vi "Labview Hardware Config file read key.vi"(5 "error in (no error)":errorcluster, 6 "Interactive?":bool=TRUE, 7 "key name in":string="Port", 8 "section":string="Panasonic AG7300") -> (0 "error out":errorcluster, 1 "File read":path, 3 "key vlue out":string)   [LabVIEW 2016]
uses:
  <vilib>/Utility/config.llb/NI_LVConfig.lvlib
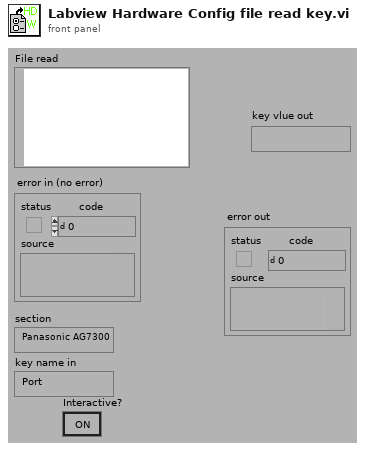
[diagram p1: front panel]
types:
  T1 = typedef "NI_LVConfig.lvlib/Config Data RefNum.ctl" = refnum<k1>
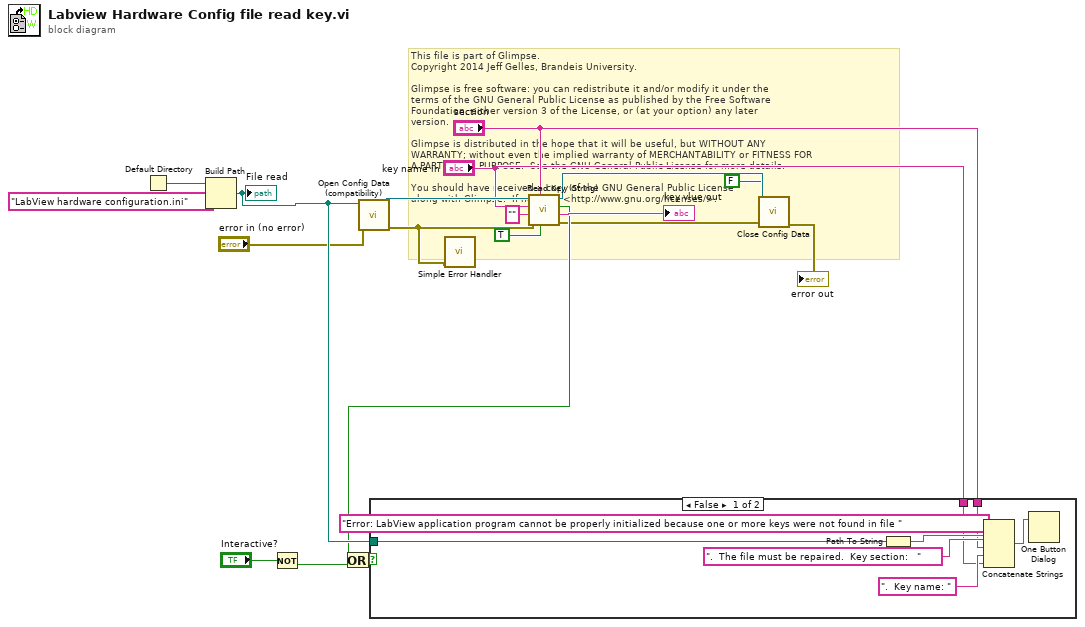
[diagram p0: block diagram]
diagram:
  # "This file is part of Glimpse. \nCopyright 2014 Jeff Gelles, Brandeis University.    \n\nGlimpse is free software: you can redistribute it and/or modify it under the \nterms of the GNU General Public License as published by the Free Software \nFoundation, either version 3 of the License, or (at your option) any later \nversion.\n\nGlimpse is distributed in the hope that it will be useful, but WITHOUT ANY \nWARRANTY; without even the implied warranty of MERCHANTABILITY or FITNESS FOR \nA PARTICULAR PURPOSE.  See the GNU General Public License for more details.\n\nYou should have received a copy of the GNU General Public License\nalong with Glimpse.  If not, see <http://www.gnu.org/licenses/>."
  n1 = Default Directory() -> (w18:path)
  n2 = Build Path(base path=w18, name or relative path="LabView hardware configuration.ini") -> (appended path=w15:path)
  "File read" <- w15
  n3 = Not(x="Interactive?") -> (.not. x?=w2:bool)
  n4 = call <vilib>:"Open Config Data (compatibility).vi"("error in (no error)"="error in (no error)", "configuration file path"=w15) -> ("error out"=w13:errorcluster, "refnum"=w17:T1)  [unwired: 7 in, 1 out]
  n5 = call <vilib>:"Simple Error Handler.vi"("error in (no error)"=w13) -> ()  [unwired: 1 in, 8 out]
  n6 = call <vilib>:"Read Key (String).vi"("read raw string? (F)"=TRUE, "section"="section", "error in (no error)"=w13, "default value"="", "key"="key name in", "refnum"=w17) -> ("error out"=w6:errorcluster, "value"=→"key vlue out":string, "found?"=w10:bool, "refnum out"=w5:T1)  [unwired: 2 out]
  n7 = Or(x=w10, y=w2) -> (x .or. y?=w4:bool)
  n8 = case shown="False" w4 {
    tunnel: w15 -> [w26 _]
    tunnel: "section" -> [w21 _]
    tunnel: "key name in" -> [w20 _]
    frame False {
      n9 = Path To String(path=w26) -> (string=w25:string)
      n10 = Concatenate Strings("Error: LabView application program cannot be properly initialized because one or more keys were not found in file " ("Substring"), w25, ".  The file must be repaired.  Key section:   " ("Substring"), w21, ".  Key name: " ("string"), w20) -> (w24:string)
      n11 = One Button Dialog(message=w24) -> ()  [unwired: 2 out]
    }
    frame True {
    }
  }
  n12 = call <vilib>:"Close Config Data.vi"("error in (no error)"=w6, "write file if changed (T)"=FALSE ("write configuration file? (T)"), "refnum"=w5) -> ("error out"=→"error out":errorcluster)  [unwired: 8 out]
